vi "insert text to pic.vi"(10 "BlueChannel in":u8[](array[numeric]), 11 "Path":path) -> (2 "BlueChannel out(textData)":u8[](array[numeric]), 3 "String":string)   [LabVIEW 2016]
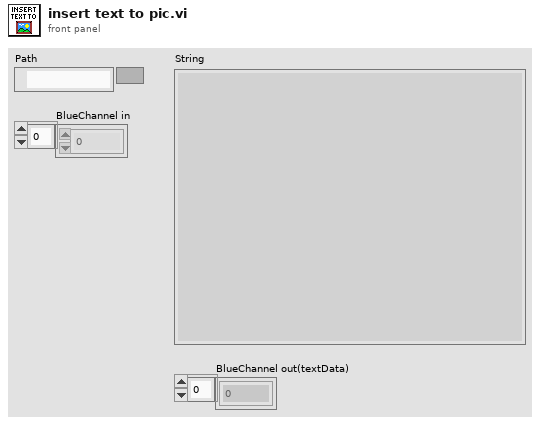
[diagram p1: front panel]
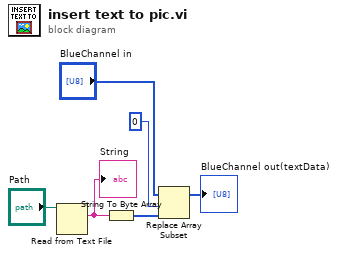
[diagram p0: block diagram]
diagram:
  n1 = Read from Text File(file (use dialog)="Path") -> (text=w2:string)  [unwired: 3 in, 3 out]
  "String" <- w2
  n2 = String To Byte Array(string=w2) -> (unsigned byte array=w3:u8[])
  n3 = Replace Array Subset(array="BlueChannel in", new element=w3, index=0) -> (→"BlueChannel out(textData)":u8[])
